vi "yytest.vi"() -> ()   [LabVIEW 2012]
panel:
  in  "string":string="QAMT06\\CRH3605"
  out "error out":errorcluster
  out "element":string
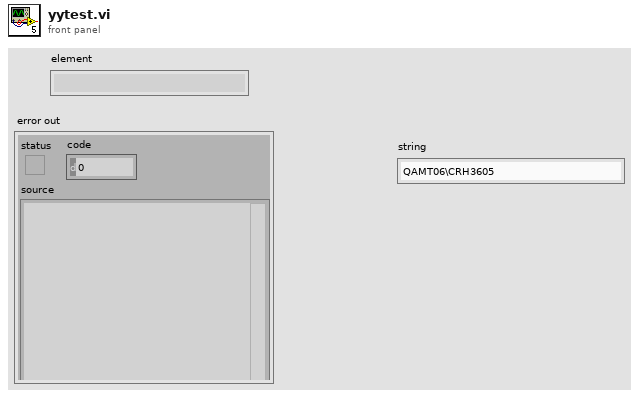
[diagram p1: front panel]
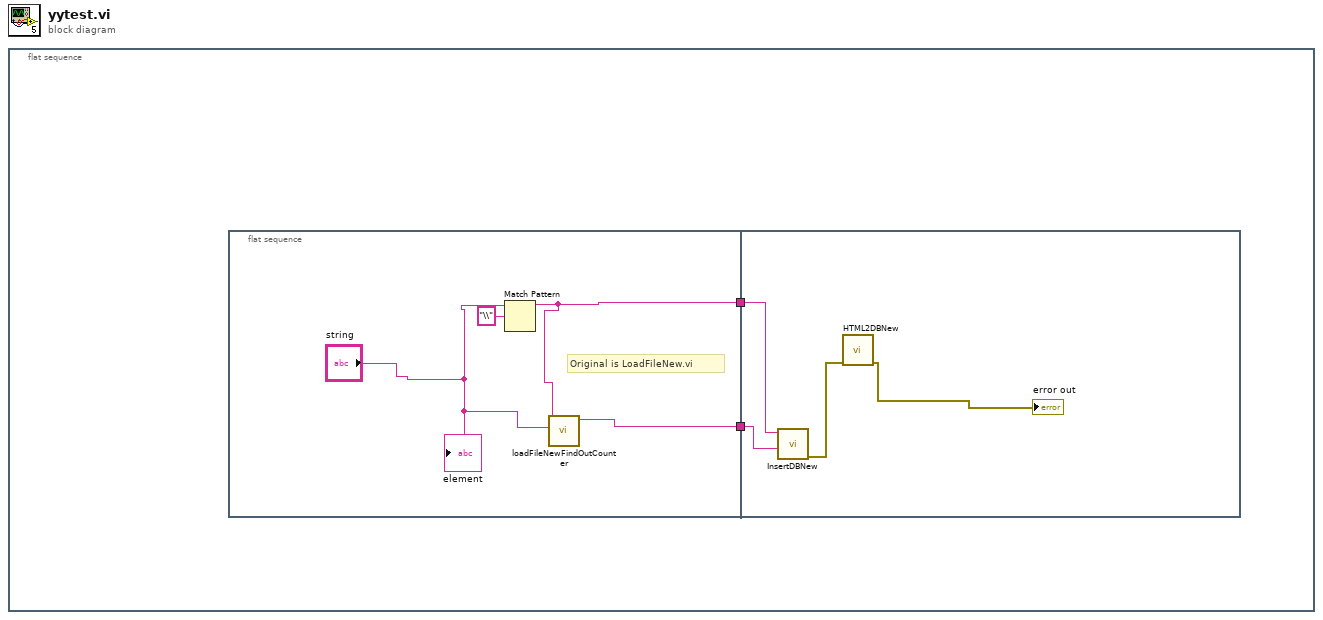
[diagram p0: block diagram]
diagram:
  n1 = flat-sequence {
    frame #0 {
      n2 = flat-sequence {
        tunnel: [w5] -> w2
        tunnel: [w3] -> w1
        tunnel: w2 -> [w9]
        tunnel: w1 -> [w8]
        frame #0 {
          # "Original is LoadFileNew.vi"
          n3 = Match Pattern(string="string", regular expression="\\") -> (before substring=w3:string)  [unwired: 1 in, 3 out]
          n4 = call "loadFileNewFindOutCounter.vi"("folder"="string", "Entity"=w3) -> ("Lot"=w5:string)  [unwired: 8 in, 1 out]
          "element" <- "string"
        }
        frame #1 {
          n5 = call "InsertDBNew.vi"("String"=w9, "Entity"=w8) -> ("error out"=w10:errorcluster)  [unwired: 9 in]
          n6 = call "HTML2DBNew.vi"("error in (no error)"=w10) -> ("error out"=→"error out":errorcluster)  [unwired: 10 in]
        }
      }
    }
  }
